vi "Actor Core.vi"(8 "error in":errorcluster, 11 "Main ViewManager In":refnum<class "Main ViewManager.lvclass">) -> (0 "error out":errorcluster, 3 "Actor out":refnum<class "Actor.lvclass">)   [LabVIEW 2019, in "Main ViewManager.lvclass"]
doc: "(<B>Filename</B>: Actor Framework.lvlib:Actor.lvclass:Actor Core.vi)\n\nReceives messages to the actor, reacts to them, and initiates any error handling that may shut the actor down.\n\nDescendant classes may override this VI to append parallel tasks for the actor to complete while it handles messages. Overrides use the Call Parent Method node.\n\n<License>\nCopyright © 2017 Composed Systems, LLC | All rights reserved\nwww.composed.io\n\nAuthor: Ethan Stern <ethan.stern@composed.io>\n\nThis software is provided \"AS IS\" WITHOUT WARRANTIES, either express or implied, AND IS FOR EDUCATIONAL PURPOSES ONLY.\n</License>"
uses:
  <vilib>/gpm_packages/@cs/Car-wash/Source/Main ViewManager/Main ViewManager/Main ViewManager.lvclass
  <vilib>/gpm_packages/@cs/mva-viewable/Source/IViewable/ProtectedSubpanel/ProtectedSubpanel.lvclass
  <vilib>/gpm_packages/@cs/mva-viewable/Source/IViewManager/IViewManager/IViewManager.lvclass
  <vilib>/ActorFramework/Actor/Actor.lvclass
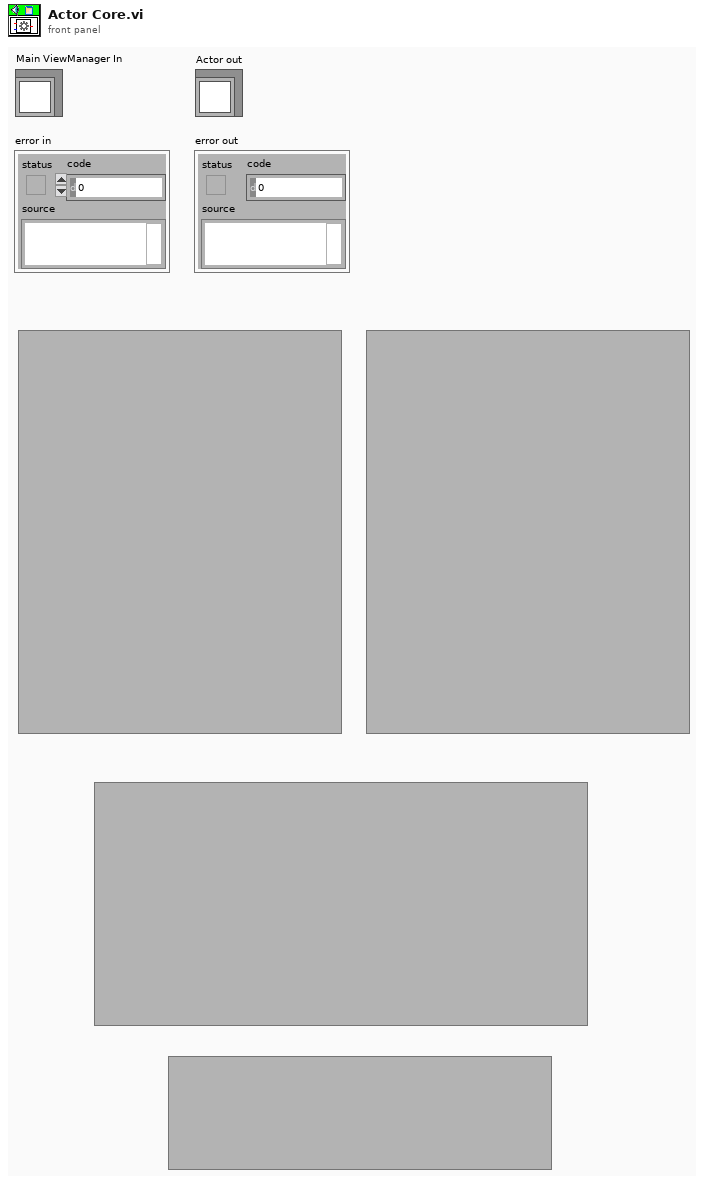
[diagram p1: front panel]
types:
  T1 = typedef "IViewable.lvlib/ProtectedSubpanel.lvclass/Protected Subpanel Reference.ctl" = refnum<data-value>
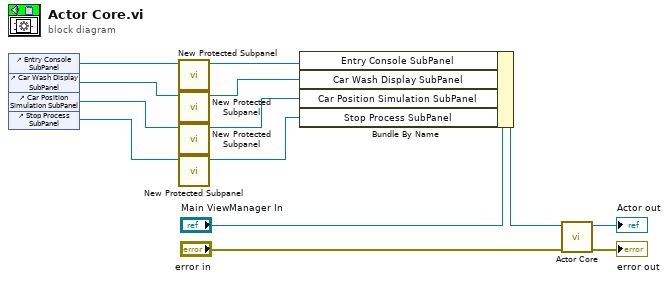
[diagram p0: block diagram]
diagram:
  n1 = control-ref of="Entry Console SubPanel"() -> (w9:refnum<vi>)
  n2 = control-ref of="Car Wash Display SubPanel"() -> (w10:refnum<vi>)
  n3 = control-ref of="Car Position Simulation SubPanel"() -> (w11:refnum<vi>)
  n4 = control-ref of="Stop Process SubPanel"() -> (w4:refnum<vi>)
  n5 = call <vilib>:"New Protected Subpanel.vi"("SubPnl Refnum"=w9) -> ("Protected Subpanel"=w8:T1)  [unwired: 9 in, 1 out]
  n6 = call <vilib>:"New Protected Subpanel.vi"("SubPnl Refnum"=w10) -> ("Protected Subpanel"=w7:T1)  [unwired: 9 in, 1 out]
  n7 = call <vilib>:"New Protected Subpanel.vi"("SubPnl Refnum"=w11) -> ("Protected Subpanel"=w6:T1)  [unwired: 9 in, 1 out]
  n8 = call <vilib>:"New Protected Subpanel.vi"("SubPnl Refnum"=w4) -> ("Protected Subpanel"=w3:T1)  [unwired: 9 in, 1 out]
  n9 = Bundle By Name(cluster="Main ViewManager In", "Entry Console SubPanel"=w8, "Car Wash Display SubPanel"=w7, "Car Position Simulation SubPanel"=w6, "Stop Process SubPanel"=w3) -> (w1:refnum<class "Main ViewManager.lvclass">)
  n10 = call-parent "Actor Core.vi"("error in"="error in", "IViewable In"=w1) -> ("error out"=→"error out":errorcluster, "Actor out"=→"Actor out":refnum<class "Actor.lvclass">)  [unwired: 8 in]
